vi "Show View.vi"(8 "error in (no error)":errorcluster, 9 "Custom Position":cluster{"Top":i16, "Left":i16}, 10 "Position":T1, 11 "IViewable in":refnum<class "IViewable.lvclass">) -> (0 "error out":errorcluster, 3 "IViewable out":refnum<class "IViewable.lvclass">)   [LabVIEW 2015, in "IViewable.lvlib" / "IViewable.lvclass"]
uses:
  IViewable.lvclass
  View Position Enum.ctl
  IViewable.lvclass/IViewable.ctl
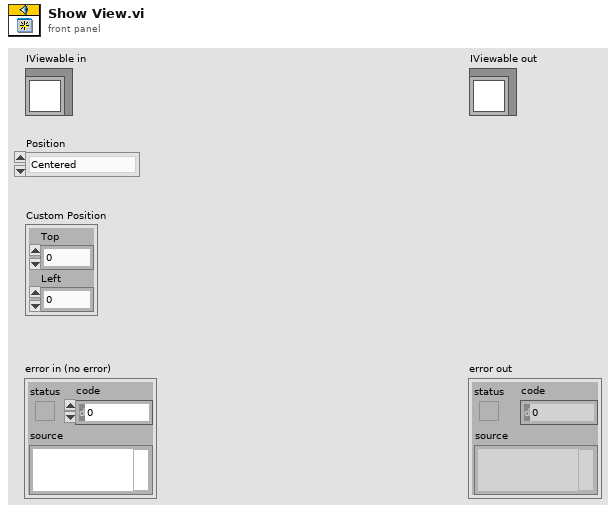
[diagram p1: front panel]
types:
  T1 = typedef "IViewable.lvlib/IViewable.lvclass/View Position Enum.ctl" = enum16{"Centered", "Maximized", "Minimized", "Custom", "Unchanged"}
  T2 = enum32{"Invalid", "Standard", "Closed", "Hidden", "Minimized", "Maximized"}
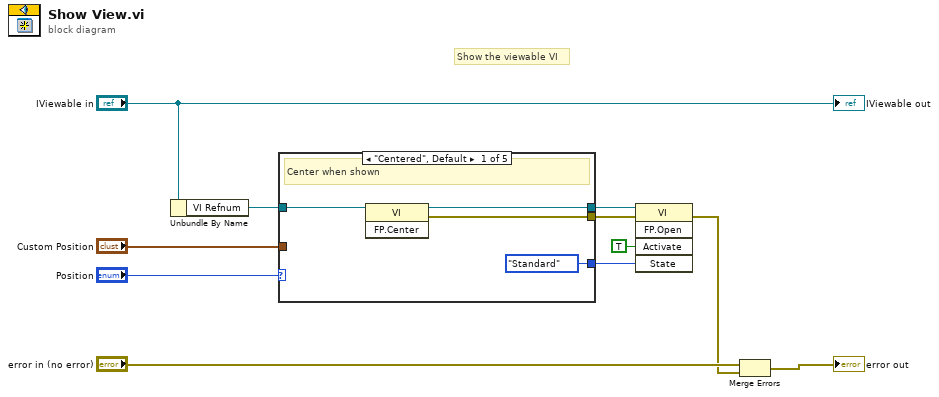
[diagram p0: block diagram]
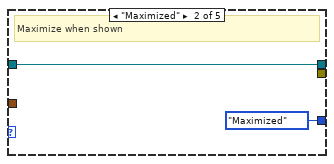
[diagram p2: hidden frame]
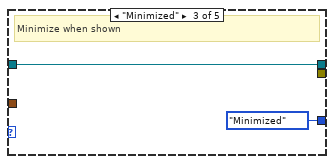
[diagram p3: hidden frame]
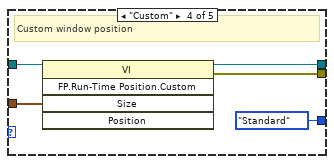
[diagram p4: hidden frame]
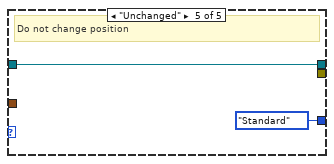
[diagram p5: hidden frame]
diagram:
  # "Show the viewable VI"
  n1 = Unbundle By Name("IViewable in") -> ("VI Refnum"=w8:refnum<vi>)
  n2 = case shown="\"Centered\", Default" "Position" {
    tunnel: w8 -> [w15 w17 w19 w24 w26]
    tunnel: [w14 w17 w19 w23 w26] -> w4
    tunnel: [w13 _ _ w22 _] -> w3
    tunnel: "Custom Position" -> [_ _ _ w21 _]
    tunnel: [T2."Standard" ("State") T2."Maximized" ("State") T2."Minimized" ("State") T2."Standard" ("State") T2."Standard" ("State")] -> w1
    frame "Centered", Default {
      # "Center when shown"
      n3 = invoke class="VI" method="FP.Center"(reference=w15) -> (reference out=w14:refnum<vi>, error out=w13:errorcluster)  [unwired: 2 in, 1 out]
    }
    frame "Maximized" {
      # "Maximize when shown"
    }
    frame "Minimized" {
      # "Minimize when shown"
    }
    frame "Custom" {
      # "Custom window position"
      n4 = invoke class="VI" method="FP.Run-Time Position.Custom"(reference=w24, "Size"=w21) -> (reference out=w23:refnum<vi>, error out=w22:errorcluster)  [unwired: 3 in, 3 out]
    }
    frame "Unchanged" {
      # "Do not change position"
    }
  }
  n5 = invoke class="VI" method="FP.Open"(reference=w4, error in=w3, "Activate"=TRUE ("Activate?"), "State"=w1) -> (error out=w7:errorcluster)  [unwired: 1 in, 4 out]
  n6 = Merge Errors("error in (no error)", w7) -> (→"error out":errorcluster)
  "IViewable out" <- "IViewable in"
